vi "Zamojski_10_target_2.vi"   [LabVIEW 2020]
uses:
  <vilib>/Platform/TimedLoop/XDataNode/timing_clust.ctl
  <vilib>/Platform/TimedLoop/XDataNode/nitl_modes.ctl
  <vilib>/Platform/TimedLoop/XDataNode/wakeup.ctl
  <vilib>/Platform/TimedLoop/scheduler/LVUserAPI/_suppVIs/Create_1MHz_TSource.vi
  <vilib>/platform/TimedLoop/XDataNode/XDataNode.xnode
  <vilib>/Platform/TimedLoop/XDataNode/XDNodeRunTimeDep.lvlib
types:
  T1 = typedef "XDNodeRunTimeDep.lvlib/timing_clust.ctl" = cluster{"Expected End [f-1]":u64, "Actual End [f-1]":u64, "Finished Late? [f-1]":bool, "Expected End [i-1]":u64, "Actual End [i-1]":u64, "Finished Late? [i-1]":bool, "Expected Start [i]":u64, "Actual Start [i]":u64, "Expected Start [f]":u64, "Actual Start [f]":u64, "Source Name":string, "Structure Name":string, "Period":i64, "Deadline":i64, "Offset":i64, "Start":i64, "Priority":i32, "Timeout":i32, "Mode":T2, "Wakeup Reason":T3, "Error":errorcluster, "Source Type":string, "Secondary Source Type":string, "Global End Time":u64, "Global Start Time":u64, "Frame Duration":u64, "Iteration Duration":u64, "Assigned CPU":i32, "I/O Scan Engine Mode":u32}
  T2 = typedef "XDNodeRunTimeDep.lvlib/nitl_modes.ctl" = enum32{"No Change", "Process missed periods, maintain original phase", "Discard missed periods, maintain original phase", "Process missed periods, ignore original phase", "Discard missed periods, ignore original phase"}
  T3 = typedef "XDNodeRunTimeDep.lvlib/wakeup.ctl" = enum32{"Normal", "Aborted", "Asynchronous wakeup", "Timing source error", "Timed loop error", "Timeout"}
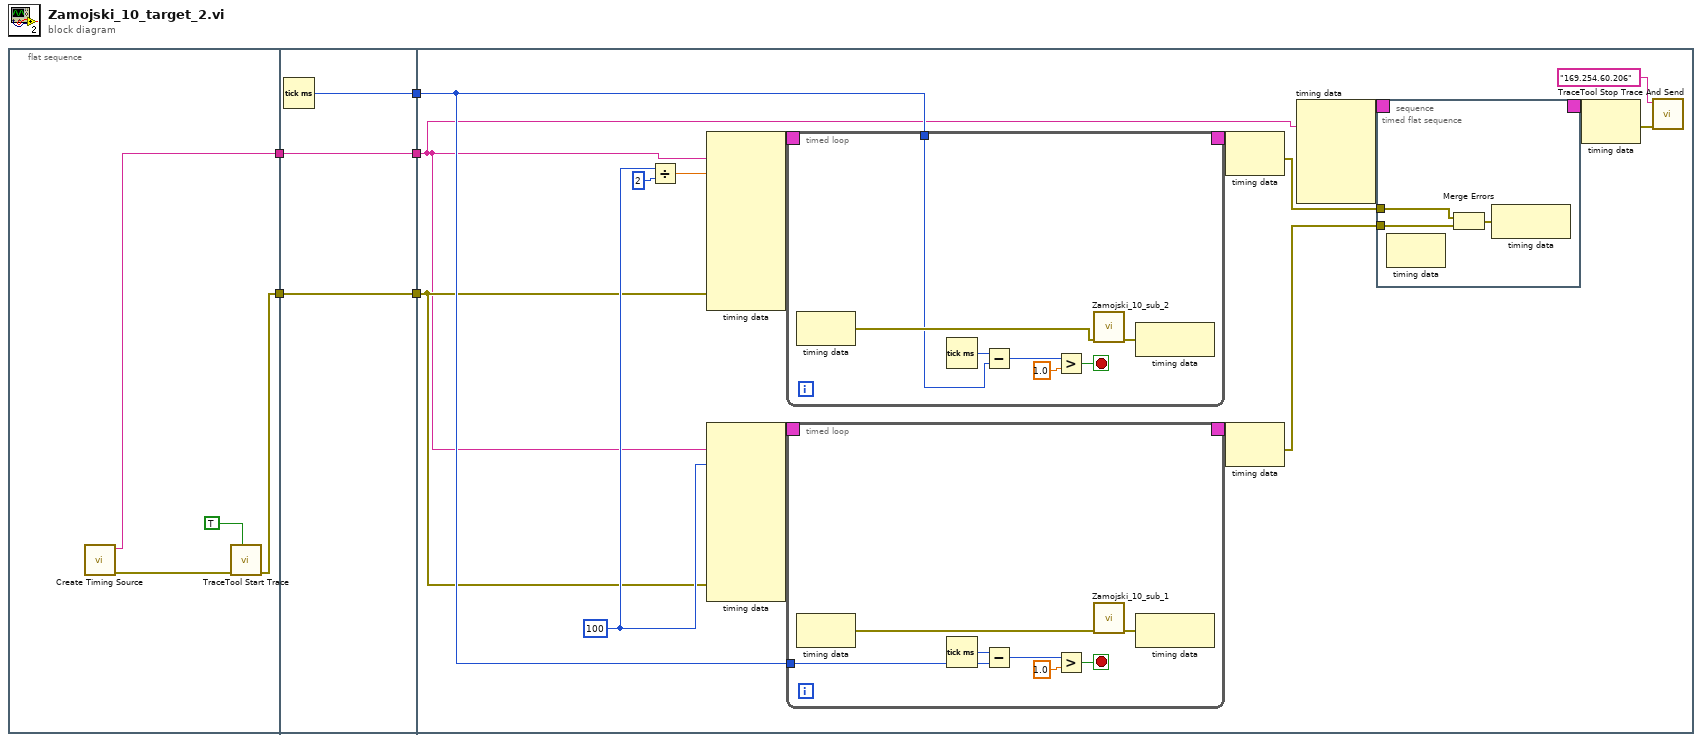
[diagram p0: block diagram]
diagram:
  n1 = flat-sequence {
    tunnel: [w7] -> w3
    tunnel: [w6] -> w1
    tunnel: [w12] -> w5
    tunnel: [w11] -> w4
    tunnel: w3 -> [w11]
    tunnel: [w10] -> w2
    tunnel: w1 -> [w10]
    tunnel: w5 -> [w15]
    tunnel: w4 -> [w14]
    tunnel: w2 -> [w13]
    frame #0 {
      n2 = call-poly <vilib>:"Create Timing Source.vi"() -> ("error out"=w9:errorcluster, "name (out)"=w6:string)  [unwired: 10 in]
      n3 = call <vilib>:"TraceTool Start Trace.vi"("Detailed Tracing? (F)"=TRUE, "error in (no error)"=w9) -> ("error out"=w7:errorcluster)  [unwired: 8 in, 1 out]
    }
    frame #1 {
      n4 = Tick Count (ms)() -> (millisecond timer value=w12:u32)
    }
    frame #2 {
      w19 = i64 100 ("Period")
      n5 = Divide(x=w19, y=i64 2) -> (x/y=w20:dbl)
      n6 = node-c288(w13, w20, w14) -> (w22:T1)  [unwired: 7 in]
      n7 = node-c288(w13, w19, w14) -> (w28:T1)  [unwired: 7 in]
      n8 = timed-loop {
        timing: w22 -> [_]
        timing-out: [_] -> w21
        tunnel: w15 -> [w29]
        stop <- w33 stop-if-true
        n9 = node-c288() -> (w32:errorcluster)  [unwired: 1 in]
        n10 = Tick Count (ms)() -> (millisecond timer value=w30:u32)
        n11 = Subtract(x=w30, y=w29) -> (x-y=w34:u32)
        n12 = Greater?(x=w34, y=1.0) -> (0:w33:bool)
        n13 = call "Zamojski_10_sub_2.vi"("error in (no error)"=w32) -> ("error out"=w31:errorcluster)  [unwired: 10 in]
        n14 = node-c288(w31) -> ()  [unwired: 1 out]
      }
      n15 = timed-loop {
        timing: w28 -> [_]
        timing-out: [_] -> w27
        tunnel: w15 -> [w62]
        stop <- w66 stop-if-true
        n16 = node-c288() -> (w65:errorcluster)  [unwired: 1 in]
        n17 = Tick Count (ms)() -> (millisecond timer value=w63:u32)
        n18 = Subtract(x=w63, y=w62) -> (x-y=w68:u32)
        n19 = Greater?(x=w68, y=1.0) -> (0:w66:bool)
        n20 = call "Zamojski_10_sub_1.vi"("error in (no error)"=w65) -> ("error out"=w64:errorcluster)  [unwired: 10 in]
        n21 = node-c288(w64) -> ()  [unwired: 1 out]
      }
      n22 = node-c288(w21) -> (w16:errorcluster)
      n23 = node-c288(w27) -> (w17:errorcluster)
      n24 = node-c288(w13) -> (w26:T1)  [unwired: 4 in]
      n25 = timed-sequence {
        timing: w26 -> [_]
        timing-out: [_] -> w25
        tunnel: w17 -> [w49]
        tunnel: w16 -> [w48]
        n26 = timed-flat-sequence {
          tunnel: w49 -> [w52]
          tunnel: w48 -> [w51]
          n27 = node-c288() -> ()  [unwired: 1 in, 1 out]
          n28 = Merge Errors(w51, w52) -> (w50:errorcluster)
          n29 = node-c288(w50) -> ()  [unwired: 1 out]
        }
      }
      n30 = node-c288(w25) -> (w24:errorcluster)
      n31 = call <vilib>:"TraceTool Stop Trace And Send.vi"("error in (no error)"=w24, "Trace Host Network Address"="169.254.60.206") -> ()  [unwired: 9 in, 1 out]
    }
  }
